vi "AccelerometerDataLoop.vi"   [LabVIEW 2016]
uses:
  Telemetry/TelemetryDataTypes.ctl
  Telemetry/TelemetryUpdateModes.ctl
  Telemetry/TelemetryFields.ctl
  <vilib>/rvi/Emulation/niFpgaGetClockAttributes.vi
  <vilib>/rvi/Emulation/niFpgaSctlEmulationGetInTimedLoop.vi
  <vilib>/rvi/Emulation/niFpgaEmulationReportErrorSimple.vi
  <vilib>/rvi/Emulation/niFpgaEmulationIsFPGAContextNoSignature.vi
  <vilib>/rvi/errors/niFpgaSetErrorForExecOnDevCompSimple.vi
  <vilib>/rvi/eio/common/nirviEmuReportErrorAndStop.vi
  <vilib>/rvi/DataTransferAndStorage/Container/Common/niFpgaContainerGetUniqueNameForEmu.vi
  <vilib>/rvi/FIFO/Fifo_Resource/nirvififoEmulationSetSize.vi
  <vilib>/rvi/FIFO/Fifo_Resource/nirviFifoEmulationQueueMgr.vi
  <instcachedir>/0/nirviFifoEmulationQueueMgr_E5CAEC123FF24DC58D834DCA3CDAA9B5.lvgen/nirviFifoEmulationQueueMgr_E5CAEC123FF24DC58D834DCA3CDAA9B5_026.vi
  <vilib>/Utility/error.llb/Clear Errors.vi
  <vilib>/rvi/FIFO/Fifo_Resource/nirvififoEmulationCreateLock.vi
  <vilib>/rvi/Emulation/niFpgaProcessEmulError.vi
  <vilib>/rvi/FIFO/Fifo_Resource/nirvififoEmulationObtainLock.vi
  <vilib>/rvi/FIFO/Fifo_Resource/nirvififoEmulationReleaseLock.vi
  <vilib>/rvi/occurrence/nirviWaitOnOccurrenceBase.vi
  <vilib>/rvi/errors/nirviReportUnexpectedCaseInternalError.vi
  <vilib>/rvi/errors/nirviReportUnexpectedCaseInternalError (U32).vi
  <instcachedir>/0/nirviFifoEmulationQueueMgr_E5CAEC123FF24DC58D834DCA3CDAA9B5.lvgen/nirviFifoEmulationQueueMgr_E5CAEC123FF24DC58D834DCA3CDAA9B5_024.vi
  <vilib>/rvi/FIFO/Fifo_Resource/nirvififoEmulationDetermineInputValidOut.vi
  <instcachedir>/0/nirviFifoEmulationQueueMgr_E5CAEC123FF24DC58D834DCA3CDAA9B5.lvgen/nirviFifoEmulationQueueMgr_E5CAEC123FF24DC58D834DCA3CDAA9B5_025.vi
  <instcachedir>/0/nirviFifoEmulationQueueMgr_E5CAEC123FF24DC58D834DCA3CDAA9B5.lvgen/nirviFifoEmulationQueueMgr_E5CAEC123FF24DC58D834DCA3CDAA9B5_004.vi
  <vilib>/rvi/Emulation/niFpgaCriticalErrorInLSC.vi
  <vilib>/rvi/DataTransferAndStorage/Container/XNode/niFpgaContainer.xnode
  <vilib>/rvi/FIFO/Fifo_Resource/nirvififoEmulationRead.vi
  <vilib>/rvi/FIFO/Fifo_Resource/nirvififoEmulationWrite.vi
types:
  T1 = typedef "TelemetryFields.ctl" = enum16{"InclinometerErrorCode", "InclinometerTxBytes", "InclinometerRxBytes", "InclinometerTxFrames", "InclinometerRxFrames", "InclinometerTimestamp", "InclinometerAngle", "DisplacementErrorCode", "DisplacementTxBytes", "DisplacementRxBytes", "DisplacementTxFrames", "DisplacementRxFrames", "DisplacementTimestamp", "Displacement1", "Displacement2", "Displacement3", "Displacement4", "Displacement5", "Displacement6", "Displacement7", "Displacement8", "AccelerometerSampleCount", "AccelerometerTimestamp", "AccelerometerRaw1", "AccelerometerRaw2", "AccelerometerRaw3", "AccelerometerRaw4", "AccelerometerRaw5", "AccelerometerRaw6", "AccelerometerRaw7", "AccelerometerRaw8", "AccelerometerEng1", "AccelerometerEng2", "AccelerometerEng3", "AccelerometerEng4", "AccelerometerEng5", "AccelerometerEng6", "AccelerometerEng7", "AccelerometerEng8", "AngularAccelerationX", "AngularAccelerationY", "AngularAccelerationZ"}
  T2 = typedef "TelemetryUpdateModes.ctl" = enum8{"=", "+", "-", "|"}
  T3 = typedef "TelemetryDataTypes.ctl" = enum8{"U8", "U16", "U32", "U64", "I8", "I16", "I32", "I64", "SGL"}
  T4 = cluster{"Timestamp":u64, "Accelerometer1Voltage":sgl, "Accelerometer2Voltage":sgl, "Accelerometer3Voltage":sgl, "Accelerometer4Voltage":sgl, "Accelerometer5Voltage":sgl, "Accelerometer6Voltage":sgl, "Accelerometer7Voltage":sgl, "Accelerometer8Voltage":sgl, "Accelerometer1Acceleration":sgl, "Accelerometer2Acceleration":sgl, "Accelerometer3Acceleration":sgl, "Accelerometer4Acceleration":sgl, "Accelerometer5Acceleration":sgl, "Accelerometer6Acceleration":sgl, "Accelerometer7Acceleration":sgl, "Accelerometer8Acceleration":sgl, "AngularAccelerationX":sgl, "AngularAccelerationY":sgl, "AngularAccelerationZ":sgl}
  T5 = typedef "TelemetryUpdateData.ctl" = cluster{"DataType":T3, "Mode":T2, "Field":T1, "Data":u64}
  T6 = typedef "TelemetryUpdateDataSGL.ctl" = cluster{"Mode":T2, "Field":T1, "Data":sgl}
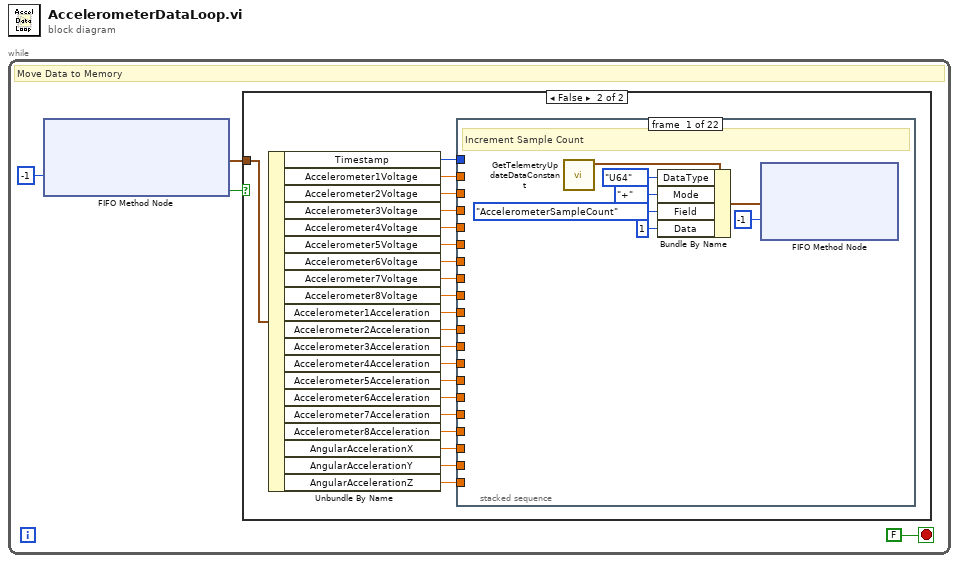
[diagram p0: block diagram]
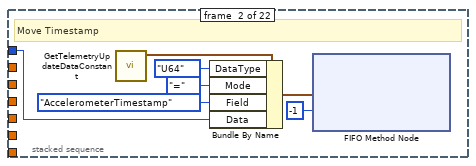
[diagram p3: hidden frame]
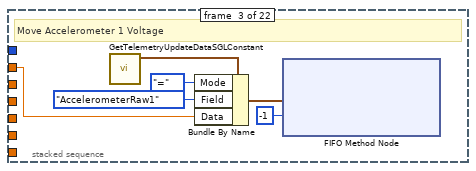
[diagram p4: hidden frame]
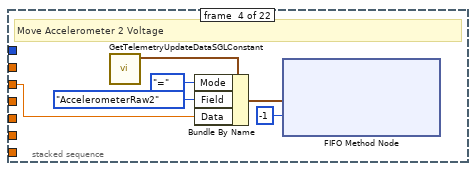
[diagram p5: hidden frame]
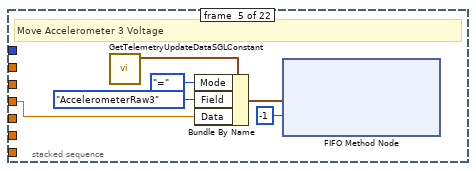
[diagram p6: hidden frame]
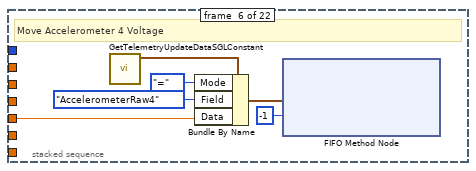
[diagram p7: hidden frame]
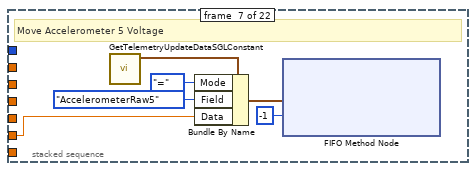
[diagram p8: hidden frame]
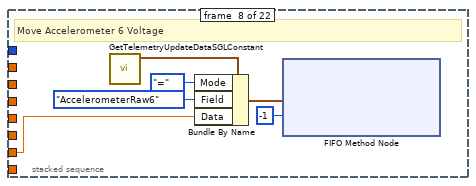
[diagram p9: hidden frame]
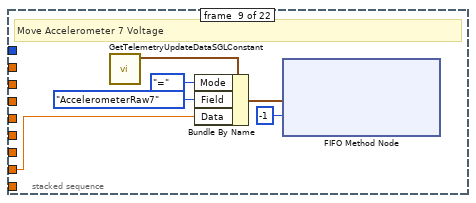
[diagram p10: hidden frame]
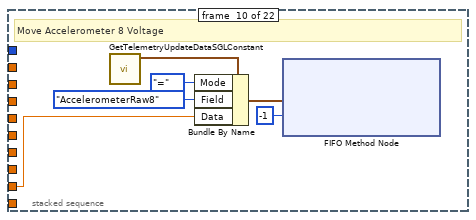
[diagram p11: hidden frame]
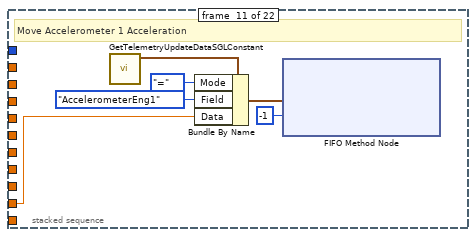
[diagram p12: hidden frame]
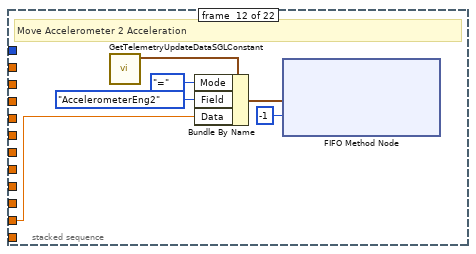
[diagram p13: hidden frame]
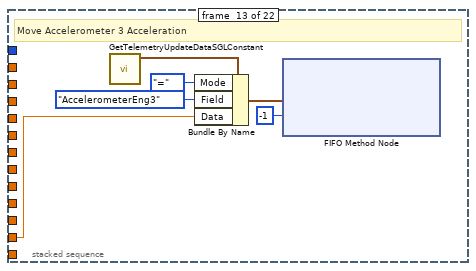
[diagram p14: hidden frame]
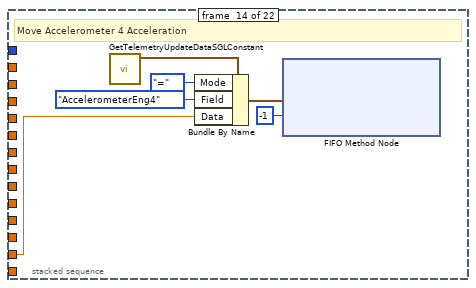
[diagram p15: hidden frame]
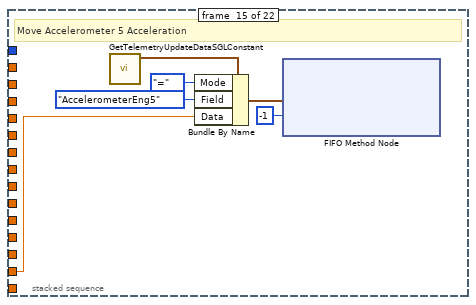
[diagram p16: hidden frame]
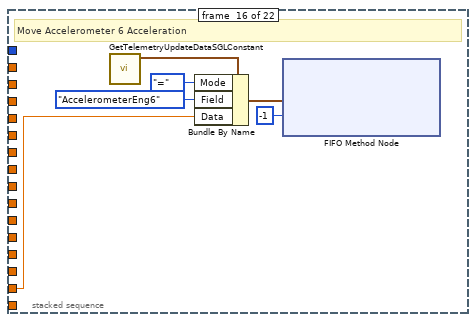
[diagram p17: hidden frame]
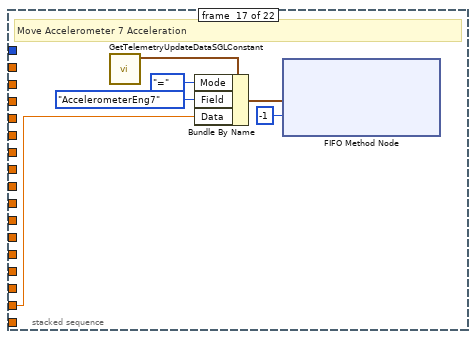
[diagram p18: hidden frame]
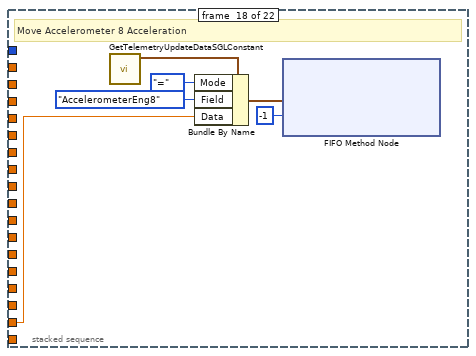
[diagram p19: hidden frame]
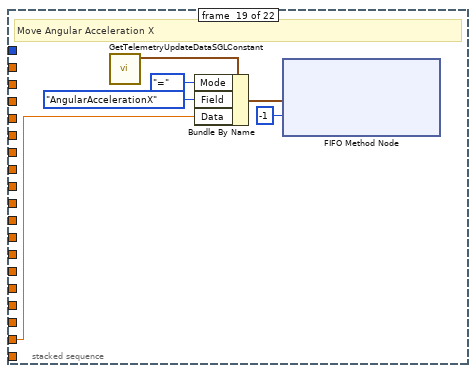
[diagram p20: hidden frame]
diagram:
  n1 = while {
    stop <- FALSE stop-if-true
    # "Move Data to Memory"
    n2 = xnode ("FIFO Method Node")("Timeout"=-1) -> ("Element"=w2:T4, "Timed Out?"=w3:bool)  [unwired: 1 in, 1 out]
    n3 = case shown="False" w3 {
      tunnel: w2 -> [_ w25]
      frame True {
      }
      frame False {
        n4 = Unbundle By Name(w25) -> ("Timestamp"=w24:u64, "Accelerometer1Voltage"=w23:sgl, "Accelerometer2Voltage"=w22:sgl, "Accelerometer3Voltage"=w21:sgl, "Accelerometer4Voltage"=w20:sgl, "Accelerometer5Voltage"=w19:sgl, "Accelerometer6Voltage"=w18:sgl, "Accelerometer7Voltage"=w17:sgl, "Accelerometer8Voltage"=w16:sgl, "Accelerometer1Acceleration"=w15:sgl, "Accelerometer2Acceleration"=w14:sgl, "Accelerometer3Acceleration"=w13:sgl, "Accelerometer4Acceleration"=w12:sgl, "Accelerometer5Acceleration"=w11:sgl, "Accelerometer6Acceleration"=w10:sgl, "Accelerometer7Acceleration"=w9:sgl, "Accelerometer8Acceleration"=w8:sgl, "AngularAccelerationX"=w7:sgl, "AngularAccelerationY"=w6:sgl, "AngularAccelerationZ"=w5:sgl)
        n5 = stacked-sequence {
          tunnel: w24 -> [_ w33 _ _ _ _ _ _ _ _ _ _ _ _ _ _ _ _ _ _ _ _]
          tunnel: w23 -> [_ _ w40 _ _ _ _ _ _ _ _ _ _ _ _ _ _ _ _ _ _ _]
          tunnel: w22 -> [_ _ _ w46 _ _ _ _ _ _ _ _ _ _ _ _ _ _ _ _ _ _]
          tunnel: w21 -> [_ _ _ _ w52 _ _ _ _ _ _ _ _ _ _ _ _ _ _ _ _ _]
          tunnel: w20 -> [_ _ _ _ _ w58 _ _ _ _ _ _ _ _ _ _ _ _ _ _ _ _]
          tunnel: w19 -> [_ _ _ _ _ _ w64 _ _ _ _ _ _ _ _ _ _ _ _ _ _ _]
          tunnel: w18 -> [_ _ _ _ _ _ _ w70 _ _ _ _ _ _ _ _ _ _ _ _ _ _]
          tunnel: w17 -> [_ _ _ _ _ _ _ _ w76 _ _ _ _ _ _ _ _ _ _ _ _ _]
          tunnel: w16 -> [_ _ _ _ _ _ _ _ _ w82 _ _ _ _ _ _ _ _ _ _ _ _]
          tunnel: w15 -> [_ _ _ _ _ _ _ _ _ _ w88 _ _ _ _ _ _ _ _ _ _ _]
          tunnel: w14 -> [_ _ _ _ _ _ _ _ _ _ _ w94 _ _ _ _ _ _ _ _ _ _]
          tunnel: w13 -> [_ _ _ _ _ _ _ _ _ _ _ _ w100 _ _ _ _ _ _ _ _ _]
          tunnel: w12 -> [_ _ _ _ _ _ _ _ _ _ _ _ _ w106 _ _ _ _ _ _ _ _]
          tunnel: w11 -> [_ _ _ _ _ _ _ _ _ _ _ _ _ _ w112 _ _ _ _ _ _ _]
          tunnel: w10 -> [_ _ _ _ _ _ _ _ _ _ _ _ _ _ _ w118 _ _ _ _ _ _]
          tunnel: w9 -> [_ _ _ _ _ _ _ _ _ _ _ _ _ _ _ _ w124 _ _ _ _ _]
          tunnel: w8 -> [_ _ _ _ _ _ _ _ _ _ _ _ _ _ _ _ _ w130 _ _ _ _]
          tunnel: w7 -> [_ _ _ _ _ _ _ _ _ _ _ _ _ _ _ _ _ _ w136 _ _ _]
          tunnel: w6 -> [_ _ _ _ _ _ _ _ _ _ _ _ _ _ _ _ _ _ _ w142 _ _]
          tunnel: w5 -> [_ _ _ _ _ _ _ _ _ _ _ _ _ _ _ _ _ _ _ _ w148 _]
          frame #0 {
            # "Increment Sample Count"
            n6 = call "GetTelemetryUpdateDataConstant.vi"() -> ("TelemetryUpdateData"=w27:T5)  [unwired: 11 in]
            n7 = Bundle By Name(cluster=w27, "DataType"=TelemetryDataTypes."U64" ("TelemetryDataTypes"), "Mode"=TelemetryUpdateModes."+" ("TelemetryUpdateModes"), "Field"=TelemetryFields."AccelerometerSampleCount" ("TelemetryFields"), "Data"=u64 1) -> (w29:T5)
            n8 = xnode ("FIFO Method Node")("Element"=w29, "Timeout"=-1) -> ()  [unwired: 1 in, 2 out]
          }
          frame #1 {
            # "Move Timestamp"
            n9 = call "GetTelemetryUpdateDataConstant.vi"() -> ("TelemetryUpdateData"=w34:T5)  [unwired: 11 in]
            n10 = Bundle By Name(cluster=w34, "DataType"=TelemetryDataTypes."U64" ("TelemetryDataTypes"), "Mode"=TelemetryUpdateModes."=" ("TelemetryUpdateModes"), "Field"=TelemetryFields."AccelerometerTimestamp" ("TelemetryFields"), "Data"=w33) -> (w36:T5)
            n11 = xnode ("FIFO Method Node")("Element"=w36, "Timeout"=-1) -> ()  [unwired: 1 in, 2 out]
          }
          frame #2 {
            # "Move Accelerometer 1 Voltage"
            n12 = call "GetTelemetryUpdateDataSGLConstant.vi"() -> ("TelemetryUpdateDataSGL"=w44:T6)  [unwired: 11 in]
            n13 = Bundle By Name(cluster=w44, "Mode"=TelemetryUpdateModes."=" ("TelemetryUpdateModes"), "Field"=TelemetryFields."AccelerometerRaw1" ("TelemetryFields"), "Data"=w40) -> (w45:T6)
            n14 = xnode ("FIFO Method Node")("Element"=w45, "Timeout"=-1) -> ()  [unwired: 1 in, 2 out]
          }
          frame #3 {
            # "Move Accelerometer 2 Voltage"
            n15 = call "GetTelemetryUpdateDataSGLConstant.vi"() -> ("TelemetryUpdateDataSGL"=w50:T6)  [unwired: 11 in]
            n16 = Bundle By Name(cluster=w50, "Mode"=TelemetryUpdateModes."=" ("TelemetryUpdateModes"), "Field"=TelemetryFields."AccelerometerRaw2" ("TelemetryFields"), "Data"=w46) -> (w51:T6)
            n17 = xnode ("FIFO Method Node")("Element"=w51, "Timeout"=-1) -> ()  [unwired: 1 in, 2 out]
          }
          frame #4 {
            # "Move Accelerometer 3 Voltage"
            n18 = call "GetTelemetryUpdateDataSGLConstant.vi"() -> ("TelemetryUpdateDataSGL"=w56:T6)  [unwired: 11 in]
            n19 = Bundle By Name(cluster=w56, "Mode"=TelemetryUpdateModes."=" ("TelemetryUpdateModes"), "Field"=TelemetryFields."AccelerometerRaw3" ("TelemetryFields"), "Data"=w52) -> (w57:T6)
            n20 = xnode ("FIFO Method Node")("Element"=w57, "Timeout"=-1) -> ()  [unwired: 1 in, 2 out]
          }
          frame #5 {
            # "Move Accelerometer 4 Voltage"
            n21 = call "GetTelemetryUpdateDataSGLConstant.vi"() -> ("TelemetryUpdateDataSGL"=w62:T6)  [unwired: 11 in]
            n22 = Bundle By Name(cluster=w62, "Mode"=TelemetryUpdateModes."=" ("TelemetryUpdateModes"), "Field"=TelemetryFields."AccelerometerRaw4" ("TelemetryFields"), "Data"=w58) -> (w63:T6)
            n23 = xnode ("FIFO Method Node")("Element"=w63, "Timeout"=-1) -> ()  [unwired: 1 in, 2 out]
          }
          frame #6 {
            # "Move Accelerometer 5 Voltage"
            n24 = call "GetTelemetryUpdateDataSGLConstant.vi"() -> ("TelemetryUpdateDataSGL"=w68:T6)  [unwired: 11 in]
            n25 = Bundle By Name(cluster=w68, "Mode"=TelemetryUpdateModes."=" ("TelemetryUpdateModes"), "Field"=TelemetryFields."AccelerometerRaw5" ("TelemetryFields"), "Data"=w64) -> (w69:T6)
            n26 = xnode ("FIFO Method Node")("Element"=w69, "Timeout"=-1) -> ()  [unwired: 1 in, 2 out]
          }
          frame #7 {
            # "Move Accelerometer 6 Voltage"
            n27 = call "GetTelemetryUpdateDataSGLConstant.vi"() -> ("TelemetryUpdateDataSGL"=w74:T6)  [unwired: 11 in]
            n28 = Bundle By Name(cluster=w74, "Mode"=TelemetryUpdateModes."=" ("TelemetryUpdateModes"), "Field"=TelemetryFields."AccelerometerRaw6" ("TelemetryFields"), "Data"=w70) -> (w75:T6)
            n29 = xnode ("FIFO Method Node")("Element"=w75, "Timeout"=-1) -> ()  [unwired: 1 in, 2 out]
          }
          frame #8 {
            # "Move Accelerometer 7 Voltage"
            n30 = call "GetTelemetryUpdateDataSGLConstant.vi"() -> ("TelemetryUpdateDataSGL"=w80:T6)  [unwired: 11 in]
            n31 = Bundle By Name(cluster=w80, "Mode"=TelemetryUpdateModes."=" ("TelemetryUpdateModes"), "Field"=TelemetryFields."AccelerometerRaw7" ("TelemetryFields"), "Data"=w76) -> (w81:T6)
            n32 = xnode ("FIFO Method Node")("Element"=w81, "Timeout"=-1) -> ()  [unwired: 1 in, 2 out]
          }
          frame #9 {
            # "Move Accelerometer 8 Voltage"
            n33 = call "GetTelemetryUpdateDataSGLConstant.vi"() -> ("TelemetryUpdateDataSGL"=w86:T6)  [unwired: 11 in]
            n34 = Bundle By Name(cluster=w86, "Mode"=TelemetryUpdateModes."=" ("TelemetryUpdateModes"), "Field"=TelemetryFields."AccelerometerRaw8" ("TelemetryFields"), "Data"=w82) -> (w87:T6)
            n35 = xnode ("FIFO Method Node")("Element"=w87, "Timeout"=-1) -> ()  [unwired: 1 in, 2 out]
          }
          frame #10 {
            # "Move Accelerometer 1 Acceleration"
            n36 = call "GetTelemetryUpdateDataSGLConstant.vi"() -> ("TelemetryUpdateDataSGL"=w92:T6)  [unwired: 11 in]
            n37 = Bundle By Name(cluster=w92, "Mode"=TelemetryUpdateModes."=" ("TelemetryUpdateModes"), "Field"=TelemetryFields."AccelerometerEng1" ("TelemetryFields"), "Data"=w88) -> (w93:T6)
            n38 = xnode ("FIFO Method Node")("Element"=w93, "Timeout"=-1) -> ()  [unwired: 1 in, 2 out]
          }
          frame #11 {
            # "Move Accelerometer 2 Acceleration"
            n39 = call "GetTelemetryUpdateDataSGLConstant.vi"() -> ("TelemetryUpdateDataSGL"=w98:T6)  [unwired: 11 in]
            n40 = Bundle By Name(cluster=w98, "Mode"=TelemetryUpdateModes."=" ("TelemetryUpdateModes"), "Field"=TelemetryFields."AccelerometerEng2" ("TelemetryFields"), "Data"=w94) -> (w99:T6)
            n41 = xnode ("FIFO Method Node")("Element"=w99, "Timeout"=-1) -> ()  [unwired: 1 in, 2 out]
          }
          frame #12 {
            # "Move Accelerometer 3 Acceleration"
            n42 = call "GetTelemetryUpdateDataSGLConstant.vi"() -> ("TelemetryUpdateDataSGL"=w104:T6)  [unwired: 11 in]
            n43 = Bundle By Name(cluster=w104, "Mode"=TelemetryUpdateModes."=" ("TelemetryUpdateModes"), "Field"=TelemetryFields."AccelerometerEng3" ("TelemetryFields"), "Data"=w100) -> (w105:T6)
            n44 = xnode ("FIFO Method Node")("Element"=w105, "Timeout"=-1) -> ()  [unwired: 1 in, 2 out]
          }
          frame #13 {
            # "Move Accelerometer 4 Acceleration"
            n45 = call "GetTelemetryUpdateDataSGLConstant.vi"() -> ("TelemetryUpdateDataSGL"=w110:T6)  [unwired: 11 in]
            n46 = Bundle By Name(cluster=w110, "Mode"=TelemetryUpdateModes."=" ("TelemetryUpdateModes"), "Field"=TelemetryFields."AccelerometerEng4" ("TelemetryFields"), "Data"=w106) -> (w111:T6)
            n47 = xnode ("FIFO Method Node")("Element"=w111, "Timeout"=-1) -> ()  [unwired: 1 in, 2 out]
          }
          frame #14 {
            # "Move Accelerometer 5 Acceleration"
            n48 = call "GetTelemetryUpdateDataSGLConstant.vi"() -> ("TelemetryUpdateDataSGL"=w116:T6)  [unwired: 11 in]
            n49 = Bundle By Name(cluster=w116, "Mode"=TelemetryUpdateModes."=" ("TelemetryUpdateModes"), "Field"=TelemetryFields."AccelerometerEng5" ("TelemetryFields"), "Data"=w112) -> (w117:T6)
            n50 = xnode ("FIFO Method Node")("Element"=w117, "Timeout"=-1) -> ()  [unwired: 1 in, 2 out]
          }
          frame #15 {
            # "Move Accelerometer 6 Acceleration"
            n51 = call "GetTelemetryUpdateDataSGLConstant.vi"() -> ("TelemetryUpdateDataSGL"=w122:T6)  [unwired: 11 in]
            n52 = Bundle By Name(cluster=w122, "Mode"=TelemetryUpdateModes."=" ("TelemetryUpdateModes"), "Field"=TelemetryFields."AccelerometerEng6" ("TelemetryFields"), "Data"=w118) -> (w123:T6)
            n53 = xnode ("FIFO Method Node")("Element"=w123, "Timeout"=-1) -> ()  [unwired: 1 in, 2 out]
          }
          frame #16 {
            # "Move Accelerometer 7 Acceleration"
            n54 = call "GetTelemetryUpdateDataSGLConstant.vi"() -> ("TelemetryUpdateDataSGL"=w128:T6)  [unwired: 11 in]
            n55 = Bundle By Name(cluster=w128, "Mode"=TelemetryUpdateModes."=" ("TelemetryUpdateModes"), "Field"=TelemetryFields."AccelerometerEng7" ("TelemetryFields"), "Data"=w124) -> (w129:T6)
            n56 = xnode ("FIFO Method Node")("Element"=w129, "Timeout"=-1) -> ()  [unwired: 1 in, 2 out]
          }
          frame #17 {
            # "Move Accelerometer 8 Acceleration"
            n57 = call "GetTelemetryUpdateDataSGLConstant.vi"() -> ("TelemetryUpdateDataSGL"=w134:T6)  [unwired: 11 in]
            n58 = Bundle By Name(cluster=w134, "Mode"=TelemetryUpdateModes."=" ("TelemetryUpdateModes"), "Field"=TelemetryFields."AccelerometerEng8" ("TelemetryFields"), "Data"=w130) -> (w135:T6)
            n59 = xnode ("FIFO Method Node")("Element"=w135, "Timeout"=-1) -> ()  [unwired: 1 in, 2 out]
          }
          frame #18 {
            # "Move Angular Acceleration X"
            n60 = call "GetTelemetryUpdateDataSGLConstant.vi"() -> ("TelemetryUpdateDataSGL"=w140:T6)  [unwired: 11 in]
            n61 = Bundle By Name(cluster=w140, "Mode"=TelemetryUpdateModes."=" ("TelemetryUpdateModes"), "Field"=TelemetryFields."AngularAccelerationX" ("TelemetryFields"), "Data"=w136) -> (w141:T6)
            n62 = xnode ("FIFO Method Node")("Element"=w141, "Timeout"=-1) -> ()  [unwired: 1 in, 2 out]
          }
          frame #19 {
            # "Move Angular Acceleration Y"
            n63 = call "GetTelemetryUpdateDataSGLConstant.vi"() -> ("TelemetryUpdateDataSGL"=w146:T6)  [unwired: 11 in]
            n64 = Bundle By Name(cluster=w146, "Mode"=TelemetryUpdateModes."=" ("TelemetryUpdateModes"), "Field"=TelemetryFields."AngularAccelerationY" ("TelemetryFields"), "Data"=w142) -> (w147:T6)
            n65 = xnode ("FIFO Method Node")("Element"=w147, "Timeout"=-1) -> ()  [unwired: 1 in, 2 out]
          }
          frame #20 {
            # "Move Angular Acceleration Z"
            n66 = call "GetTelemetryUpdateDataSGLConstant.vi"() -> ("TelemetryUpdateDataSGL"=w152:T6)  [unwired: 11 in]
            n67 = Bundle By Name(cluster=w152, "Mode"=TelemetryUpdateModes."=" ("TelemetryUpdateModes"), "Field"=TelemetryFields."AngularAccelerationZ" ("TelemetryFields"), "Data"=w148) -> (w153:T6)
            n68 = xnode ("FIFO Method Node")("Element"=w153, "Timeout"=-1) -> ()  [unwired: 1 in, 2 out]
          }
          frame #21 {
            # "Notify Processing Complete"
            n69 = xnode ("FIFO Method Node")("Element"=TRUE, "Timeout"=-1) -> ()  [unwired: 1 in, 2 out]
          }
        }
      }
    }
  }
